vi "OscCon (SubVI).vi"(8 "error in":errorcluster, 11 "A5000_param":T1={"ChannelA"={"Enabled"=FALSE, "Coupling"=1, "Range"=6, "Analogue Offset"=0.0}, "ChannelB"={"Enabled"=FALSE, "Coupling"=1, "Range"=6, "Analogue Offset"=0.0}, "Trigger"={"Trigger Enabled"=FALSE, "Trigger Source"=enum."Channel A", "Trigger Threshold (volts)"=0.0, "Trigger Direction"=2, "Trigger Delay (samples)"=0, "Auto Trigger Time (ms)"=1000}, "MaxADCvalue"=0, "handle"=0, "Acquisition"={"preTriggerSamples"=0, "postTriggerSamples"=1000, "timebase"=2, "Down-Sample Mode"=0, "Down Sample Ratio"=1}, "Device Info"={"Driver Version"="", "USB Version"="", "Hardware"="", "Variant"="", "Batch and Serial"="", "Cal Date"="", "Kernel Version"="", "Digital HW Version"="", "Analogue HW Version"="", "MSO"=FALSE, "Number of channels"=0}, "Properties"={"Sample Frequency"=0.0, "Sample Rate"=0.0, "Max Samples Available"=0, "Number of Samples"=0, "Total Capture Time (sec) "=0.0, "Max Total Capture Time Available (sec)"=0.0}, "Resolution"=3, "EmulateV"=FALSE, "General AWG Settings"={"Peak-to-Peak Voltage (microvolts)"=2000000, "Offset Voltage (microvolts)"=0, "Wave Type"=0, "Sweep Type"=0, "Shots"=0, "Sweeps"=0, "Trigger Type"=0, "Trigger Source"=0, "Ext. Threshold (ADC count)"=0, "White Noise/PRBS"=0}, "Standard Waveform Settings"={"Start Frequency"=1000.0, "Stop Frequency"=1000.0, "Increment"=0.0, "Dwell Time (seconds)"=0.0}, "Arbitrary Waveform Settings"={"Arbirary waveform file path"=path "", "Index Mode"=0}} {"Arbitrary Waveform Settings"."Index Mode" items=["Single", "Dual", "Quad"]; "Standard Waveform Settings"."Stop Frequency" min=0.03 max=1000000.0; "Standard Waveform Settings"."Start Frequency" min=0.03 max=1000000.0; "General AWG Settings"."White Noise/PRBS" items=["Normal", "White Noise", "PRBS"]; "General AWG Settings"."Trigger Source" items=["None", "Scope Trigger", "Aux. In", "Ext. In", "Software Trigger"]; "General AWG Settings"."Trigger Type" items=["Rising", "Falling", "Gate High", "Gate Low"]; "General AWG Settings"."Sweep Type" items=["Up", "Down", "Up-Down", "Down-Up"]; "General AWG Settings"."Wave Type" items=["Sine", "Square", "Triangle", "Ramp Up", "Ramp Down", "Sinc", "Gaussian", "Half Sine", "DC", "Arbitrary"]; "Resolution" items=["8-bit", "12-bit", "14-bit", "15-bit (max. 2 ch.)", "16-bit (max. 1 ch.)"]; "Properties"."Max Total Capture Time Available (sec)" format="%.3p"; "Properties"."Sample Frequency" format="%.3p"; "Properties"."Sample Rate" format="%.3p"; "Properties"."Max Samples Available" format="%.3p"; "Properties"."Total Capture Time (sec)" format="%.3p"; "Acquisition"."Down Sample Ratio" min=1 step=1; "Acquisition"."Down-Sample Mode" items=["None"=0, "Aggregate"=1, "Decimate"=2, "Average"=4]; "Trigger"."Trigger Direction" items=["Rising"=2, "Falling"=3]; "ChannelB"."Range" items=["10 mV", "20 mV", "50 mV", "100 mV", "200 mV", "500 mV", "1 V", "2 V", "5 V", "10 V", "20 V"]; "ChannelB"."Coupling" items=["AC", "DC"]; "ChannelA"."Range" items=["10 mV", "20 mV", "50 mV", "100 mV", "200 mV", "500 mV", "1 V", "2 V", "5 V", "10 V", "20 V"]; "ChannelA"."Coupling" items=["AC", "DC"]}) -> (0 "error out":errorcluster, 2 "Connect":bool, 3 "A5000_param_out":T1={"ChannelA"={"Enabled"=FALSE, "Coupling"=1, "Range"=6, "Analogue Offset"=0.0}, "ChannelB"={"Enabled"=FALSE, "Coupling"=1, "Range"=6, "Analogue Offset"=0.0}, "Trigger"={"Trigger Enabled"=FALSE, "Trigger Source"=enum."Channel A", "Trigger Threshold (volts)"=0.0, "Trigger Direction"=2, "Trigger Delay (samples)"=0, "Auto Trigger Time (ms)"=1000}, "MaxADCvalue"=0, "handle"=0, "Acquisition"={"preTriggerSamples"=0, "postTriggerSamples"=1000, "timebase"=2, "Down-Sample Mode"=0, "Down Sample Ratio"=1}, "Device Info"={"Driver Version"="", "USB Version"="", "Hardware"="", "Variant"="", "Batch and Serial"="", "Cal Date"="", "Kernel Version"="", "Digital HW Version"="", "Analogue HW Version"="", "MSO"=FALSE, "Number of channels"=0}, "Properties"={"Sample Frequency"=0.0, "Sample Rate"=0.0, "Max Samples Available"=0, "Number of Samples"=0, "Total Capture Time (sec) "=0.0, "Max Total Capture Time Available (sec)"=0.0}, "Resolution"=0, "EmulateV"=FALSE, "General AWG Settings"={"Peak-to-Peak Voltage (microvolts)"=2000000, "Offset Voltage (microvolts)"=0, "Wave Type"=0, "Sweep Type"=0, "Shots"=0, "Sweeps"=0, "Trigger Type"=0, "Trigger Source"=0, "Ext. Threshold (ADC count)"=0, "White Noise/PRBS"=0}, "Standard Waveform Settings"={"Start Frequency"=1000.0, "Stop Frequency"=1000.0, "Increment"=0.0, "Dwell Time (seconds)"=0.0}, "Arbitrary Waveform Settings"={"Arbirary waveform file path"=path "", "Index Mode"=0}} {"Arbitrary Waveform Settings"."Index Mode" items=["Single", "Dual", "Quad"]; "Standard Waveform Settings"."Stop Frequency" min=0.03 max=1000000.0; "Standard Waveform Settings"."Start Frequency" min=0.03 max=1000000.0; "General AWG Settings"."White Noise/PRBS" items=["Normal", "White Noise", "PRBS"]; "General AWG Settings"."Trigger Source" items=["None", "Scope Trigger", "Aux. In", "Ext. In", "Software Trigger"]; "General AWG Settings"."Trigger Type" items=["Rising", "Falling", "Gate High", "Gate Low"]; "General AWG Settings"."Sweep Type" items=["Up", "Down", "Up-Down", "Down-Up"]; "General AWG Settings"."Wave Type" items=["Sine", "Square", "Triangle", "Ramp Up", "Ramp Down", "Sinc", "Gaussian", "Half Sine", "DC", "Arbitrary"]; "Resolution" items=["8-bit", "12-bit", "14-bit", "15-bit (max. 2 ch.)", "16-bit (max. 1 ch.)"]; "Properties"."Max Total Capture Time Available (sec)" format="%.3p"; "Properties"."Sample Frequency" format="%.3p"; "Properties"."Sample Rate" format="%.3p"; "Properties"."Max Samples Available" format="%.3p"; "Properties"."Total Capture Time (sec)" format="%.3p"; "Acquisition"."Down Sample Ratio" min=1 step=1; "Acquisition"."Down-Sample Mode" items=["None"=0, "Aggregate"=1, "Decimate"=2, "Average"=4]; "Trigger"."Trigger Direction" items=["Rising"=2, "Falling"=3]; "ChannelB"."Range" items=["10 mV", "20 mV", "50 mV", "100 mV", "200 mV", "500 mV", "1 V", "2 V", "5 V", "10 V", "20 V"]; "ChannelB"."Coupling" items=["AC", "DC"]; "ChannelA"."Range" items=["10 mV", "20 mV", "50 mV", "100 mV", "200 mV", "500 mV", "1 V", "2 V", "5 V", "10 V", "20 V"]; "ChannelA"."Coupling" items=["AC", "DC"]})   [LabVIEW 2017]
uses:
  controls/A5000_param.ctl
  ps5000a.dll
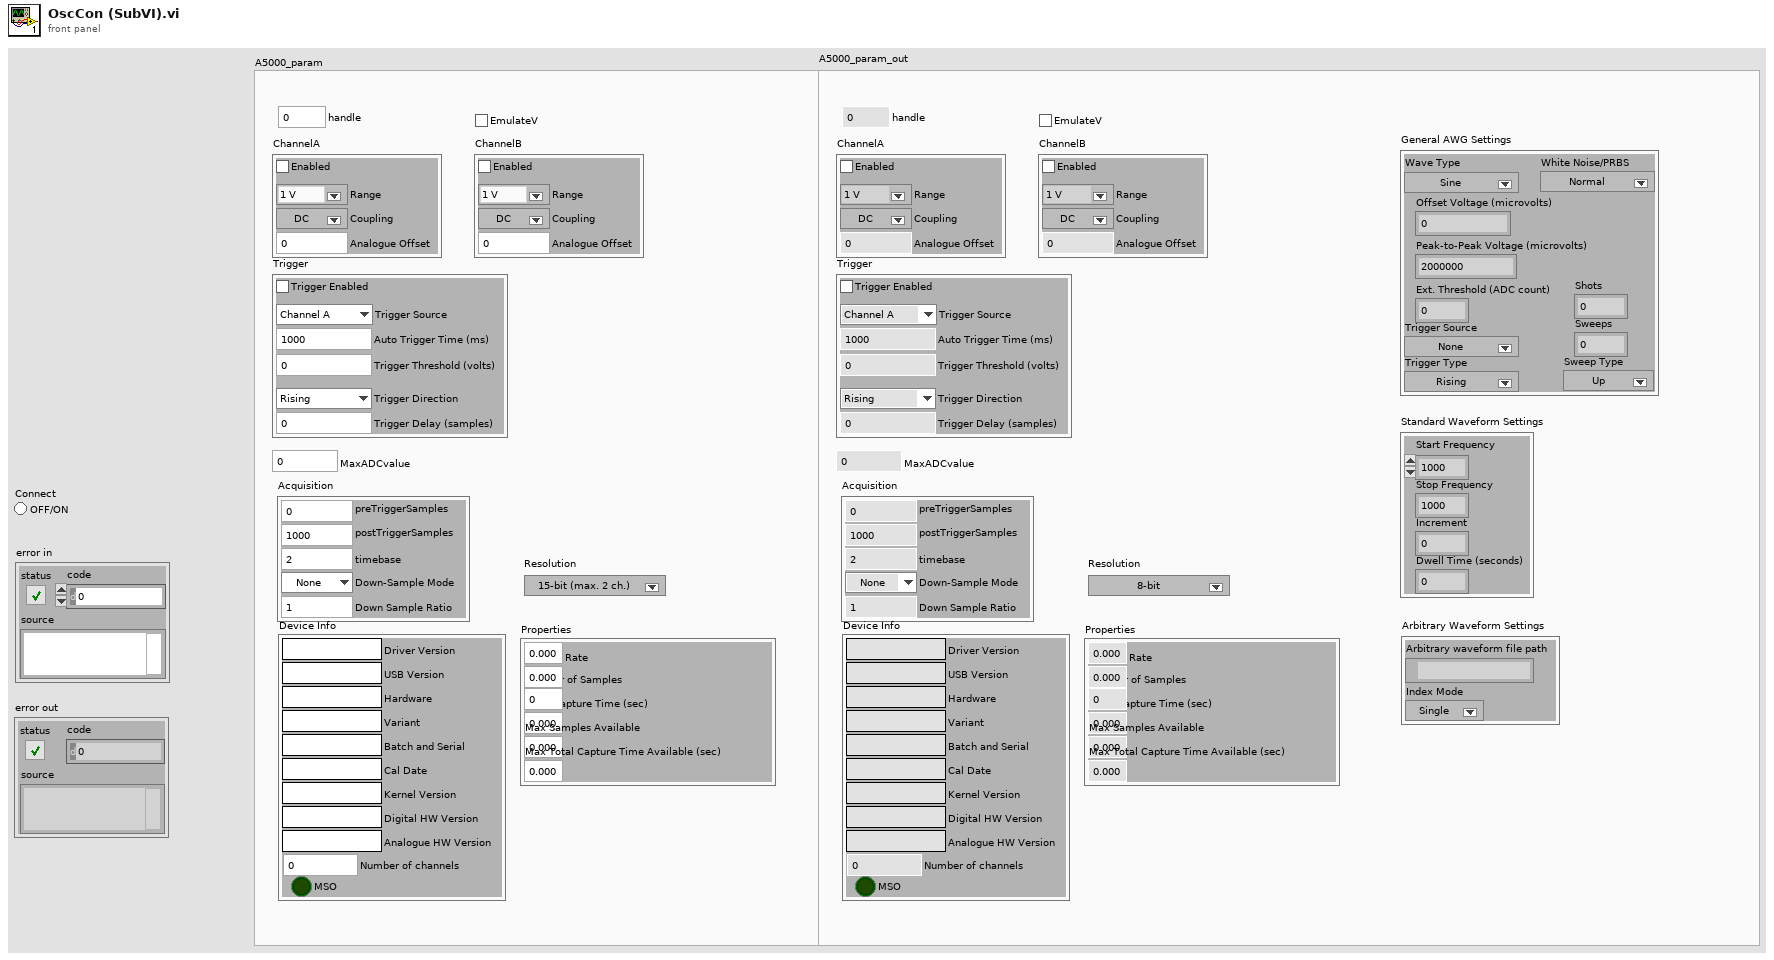
[diagram p1: front panel]
types:
  T1 = typedef "A5000_param.ctl" = cluster{"ChannelA":cluster{"Enabled":bool, "Coupling":i16, "Range":u16, "Analogue Offset":sgl}, "ChannelB":cluster{"Enabled":bool, "Coupling":i16, "Range":u16, "Analogue Offset":sgl}, "Trigger":cluster{"Trigger Enabled":bool, "Trigger Source":enum16{"Channel A", "Channel B", "Channel C", "Channel D", "Ext."}, "Trigger Threshold (volts)":dbl, "Trigger Direction":u16, "Trigger Delay (samples)":u32, "Auto Trigger Time (ms)":i16}, "MaxADCvalue":i16, "handle":i16, "Acquisition":cluster{"preTriggerSamples":i32, "postTriggerSamples":i32, "timebase":u32, "Down-Sample Mode":u32, "Down Sample Ratio":u32}, "Device Info":cluster{"Driver Version":string, "USB Version":string, "Hardware":string, "Variant":string, "Batch and Serial":string, "Cal Date":string, "Kernel Version":string, "Digital HW Version":string, "Analogue HW Version":string, "MSO":bool, "Number of channels":i16}, "Properties":cluster{"Sample Frequency":sgl, "Sample Rate":sgl, "Max Samples Available":i32, "Number of Samples":u32, "Total Capture Time (sec) ":sgl, "Max Total Capture Time Available (sec)":sgl}, "Resolution":i32, "EmulateV":bool, "General AWG Settings":cluster{"Peak-to-Peak Voltage (microvolts)":u32, "Offset Voltage (microvolts)":i32, "Wave Type":u32, "Sweep Type":u32, "Shots":u32, "Sweeps":u32, "Trigger Type":u32, "Trigger Source":u32, "Ext. Threshold (ADC count)":i16, "White Noise/PRBS":u32}, "Standard Waveform Settings":cluster{"Start Frequency":dbl, "Stop Frequency":dbl, "Increment":dbl, "Dwell Time (seconds)":dbl}, "Arbitrary Waveform Settings":cluster{"Arbirary waveform file path":path, "Index Mode":u32}}
  T2 = cluster{"Driver Version":string, "USB Version":string, "Hardware":string, "Variant":string, "Batch and Serial":string, "Cal Date":string, "Kernel Version":string, "Digital HW Version":string, "Analogue HW Version":string, "MSO":bool, "Number of channels":i16}
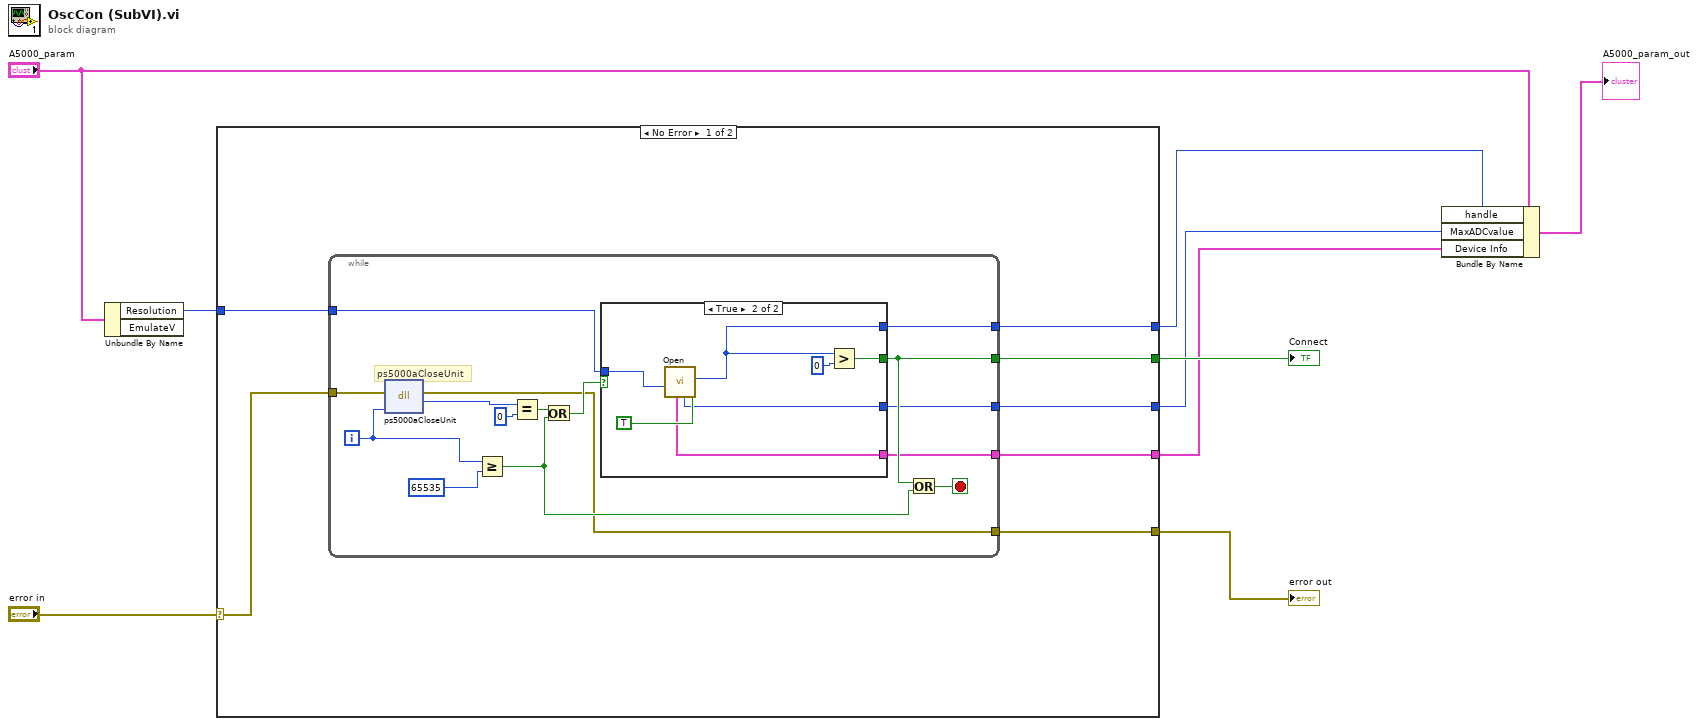
[diagram p0: block diagram]
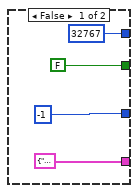
[diagram p2: hidden frame]
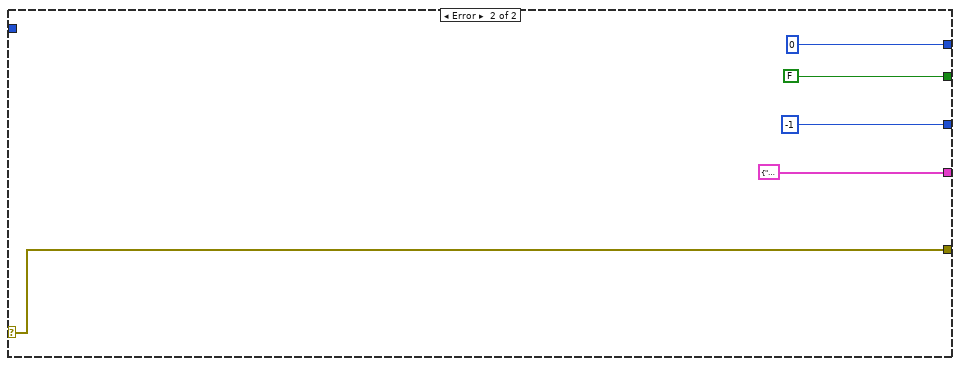
[diagram p3: hidden frame]
diagram:
  n1 = Unbundle By Name("A5000_param") -> ("Resolution"=w6:i32)  [unwired: 1 out]
  n2 = case shown="No Error" "error in" {
    selector: "error in" -> [w11 w47]
    tunnel: w6 -> [w16 _]
    tunnel: [w15 i16 0 ("handle")] -> w4
    tunnel: [w14 T2 {"Driver Version"="", "USB Version"="", "Hardware"="", "Variant"="", "Batch and Serial"="", "Cal Date"="", "Kernel Version"="", "Digital HW Version"="", "Analogue HW Version"="", "MSO"=FALSE, "Number of channels"=0} ("Device Info")] -> w2
    tunnel: [w13 i16 -1 ("Max ADC value")] -> w3
    tunnel: [w12 FALSE] -> w9
    tunnel: [w10 w47] -> w7
    frame No Error {
      n3 = while {
        tunnel: [w24] -> w12
        tunnel: [w23] -> w13
        tunnel: [w22] -> w14
        tunnel: [w21] -> w15
        tunnel: w16 -> [w19]
        tunnel: w11 -> [w18]
        tunnel: [w17] -> w10
        i -> [w31]
        stop <- w30 stop-if-true
        # "ps5000aCloseUnit"
        n4 = dll-call lib="ps5000a.dll" fn="ps5000aCloseUnit" ("ps3000.dll:_ps3000_open_unit@0")(error in=w18, "handle"=w31) -> (error out=w17:errorcluster, "PICO_STATUS"=w28:i32)  [unwired: 3 in, 1 out]
        n5 = Greater Or Equal?(x=w31, y=65535) -> (x >= y?=w20:bool)
        n6 = Equal?(x=w28, y=0) -> (x = y?=w26:bool)
        n7 = Or(x=w26, y=w20) -> (x .or. y?=w25:bool)
        n8 = case shown="True" w25 {
          tunnel: [FALSE w41] -> w24
          tunnel: [i16 -1 ("Max ADC value") w39] -> w23
          tunnel: [T2 {"Driver Version"="", "USB Version"="", "Hardware"="", "Variant"="", "Batch and Serial"="", "Cal Date"="", "Kernel Version"="", "Digital HW Version"="", "Analogue HW Version"="", "MSO"=FALSE, "Number of channels"=0} ("Device Info") w38] -> w22
          tunnel: w19 -> [_ w37]
          tunnel: [i16 32767 ("handle") w36] -> w21
          frame False {
          }
          frame True {
            n9 = call "Open.vi"("2-channel USB 3.0 device on non-USB 3.0 Port"=TRUE, "Resolution"=w37) -> ("handle"=w36:i16, "Max ADC value"=w39:i16, "Device Info"=w38:T2)  [unwired: 5 in, 2 out]
            n10 = Greater?(x=w36, y=i16 0) -> (0:w41:bool)
          }
        }
        n11 = Or(x=w24, y=w20) -> (x .or. y?=w30:bool)
      }
    }
    frame Error {
    }
  }
  "Connect" <- w9
  "error out" <- w7
  n12 = Bundle By Name(cluster="A5000_param", "handle"=w4, "MaxADCvalue"=w3, "Device Info"=w2) -> (→"A5000_param_out":T1)
